vi "DFD 2-Band Filter Bank Reconstruction.vi"   [LabVIEW 2017, in "NI_DigFilter_FilterBank.lvlib"]
doc: "Reconstructs a signal from a lowpass band signal and a highpass band signal continuously with a 2-band filter bank."
uses:
  <vilib>/addons/Digital Filter Design/NI_DigFilter_FilterBank.lvlib
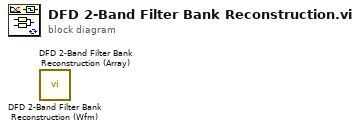
[diagram p0: block diagram]
diagram:
  n1 = call <vilib>:"DFD 2-Band Filter Bank Reconstruction (Wfm).vi"() -> ()  [unwired: 10 in, 2 out]
  n2 = call <vilib>:"DFD 2-Band Filter Bank Reconstruction (Array).vi"() -> ()  [unwired: 10 in, 2 out]
